vi "KioskDemo.vi"() -> ()   [LabVIEW 2023]
doc: "DESCRIPTION\nGeneral Application \n\nVERSION\nD1:00\nFirst Release To customer\nDD/MM/YYYY\n\nTemplate D2:01\nMade lighter and simpler\n14-04-2020"
uses:
  SubVIs/Controls/SetupModeState.ctl
  <vilib>/event_ctls.llb/eventsource.ctl
  <vilib>/Utility/miscctls.llb/LVBoundsTypeDef.ctl
  <vilib>/Utility/miscctls.llb/LVPositionTypeDef.ctl
  SubVIs/Controls/DisplayQCommand.ctl
  SubVIs/Controls/QueueCommand.ctl
  SubVIs/Controls/DisplayMessage.ctl
  SubVIs/Controls/Transition.ctl
  SubVIs/utilities/Error/ErrorCommand.ctl
  SubVIs/Controls/Tab.ctl
  SubVIs/Controls/StateMessage.ctl
  SubVIs/Error/ErrorMessage.ctl
  SubVIs/utilities/Config/System Config Data Manager Parameter.ctl
  SubVIs/utilities/Config/ConfigCommand.ctl
  SubVIs/Buttons/ButtonCommands.ctl
  SubVIs/Buttons/MenuType.ctl
panel:
  in  "ButtonsMenu":enum32{"Page 1"}(tab)
  out "SubmenuVisible":bool
  in  "Position":T1
  in  "Container Bounds":T2
  out "State":T3=enum."Initialising"
  out "UI Output":string
  out "Menu Output":string
  in  "exit":bool
  in  "Stop":bool
  in  "Source":T4 items=["LabVIEW UI"=0, "ActiveX"=1, "User Event"=25]
  out "Version":string
  out "Time":string
  in  "Main Screen Tabs":enum32{"Main Screen"}(tab)
  out "Tab Control":T5(tab)
  in  "Error Loop":enum16{"Event Loop", "UI Q Loop", "State Loop"}(ring)
  in  "Generate Error":bool
  out "EngMode?":bool
  in  "Enter Password":string
  out "ConfigdB path":path
  in  "Home Button":bool
  in  "ErrorLog":bool
  in  "Clear Alarm":bool
  in  "ErrorLog":i32(listbox)
  out "Error":string
  out "ErrorIndicator":bool
  in  "ViewError":bool
  out "Status":string
  in  "Start":bool
  out "ErrorHandlingLoop":i32
  out "StateMachineLoop":i32
  out "UILoop":i32
  out "EventLoop":i32
  # "GenAppMain"
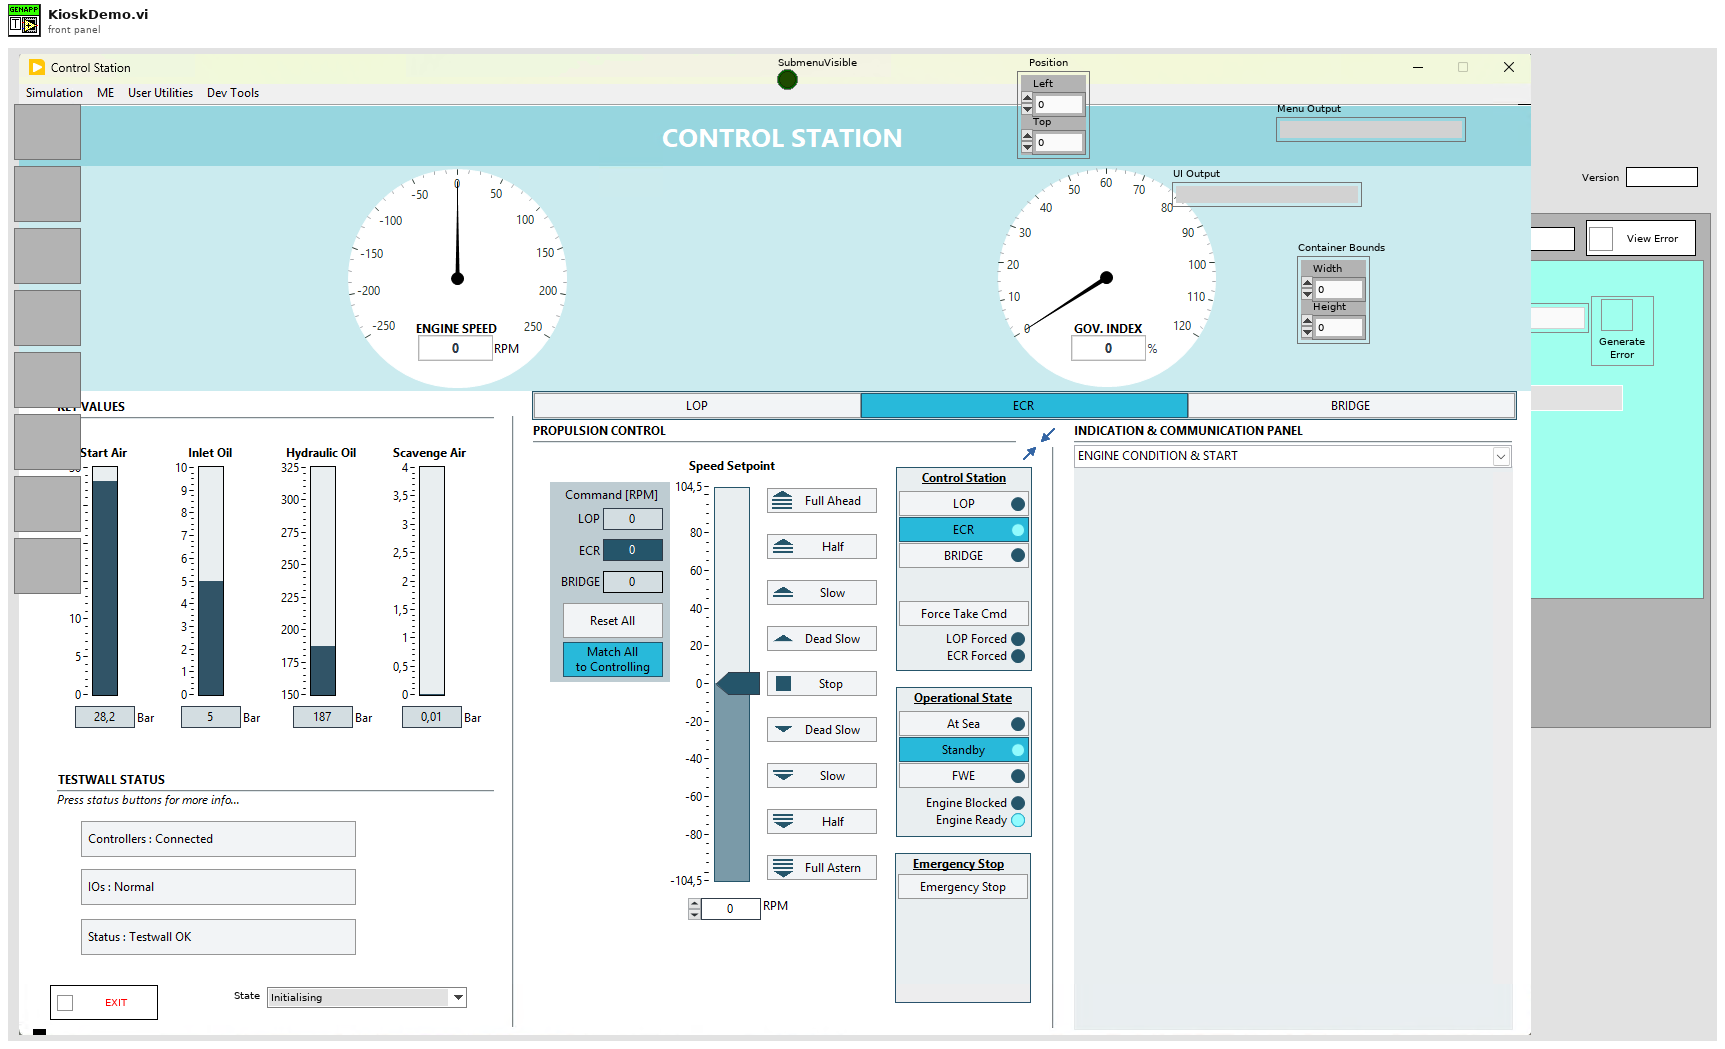
[diagram p1: front panel]
types:
  T1 = typedef "LVPositionTypeDef.ctl" = cluster{"Left":i32, "Top":i32}
  T2 = typedef "LVBoundsTypeDef.ctl" = cluster{"Width":u32, "Height":u32}
  T3 = typedef "SetupModeState.ctl" = enum16{"No State - Error", "Initialising", "Idling", "Running", "Sorting Menu", "Resetting Menu", "Loading UI", "Erroring", "Exiting"}
  T4 = typedef "eventsource.ctl" = u32
  T5 = enum32{"Welcome Screen", "Eng Set Up", "Oppo Run Screen", "Eng Run Screen", "Test Report Screen", "Error"}
  T6 = typedef "DisplayQCommand.ctl" = enum16{"No Command - Error", "Initialise", "Get Q Reference", "Add Item to Bottom", "Add Item to Top", "Flush Q", "Dequeue", "Peek Next Element", "Close"}
  T7 = typedef "QueueCommand.ctl" = enum16{"No Command - Error", "Initialise", "Add to Bottom", "Add To Top", "Get Ref", "Close"}
  T8 = typedef "ErrorCommand.ctl" = enum16{"No Command - Error", "Set to Dev Mode", "Set To Released Mode", "Set Error", "Log Error", "Throw Error", "Log & Throw Error", "Set Error Timed"}
  T9 = enum32{"invalid app kind", "Development System", "Run Time System", "Student Edition", "Embedded LabVIEW", "Evaluation", "Custom"}
  T10 = typedef "DisplayMessage.ctl" = enum16{"No Message - Ignore", "Display Message", "Set Tab", "Set Status", "Add Error Message", "Clear Error History", "Generate Error", "Set Idling Display", "Set Running Display", "Set Subpanel Output", "Stop"}
  T11 = typedef "ErrorMessage.ctl" = enum16{"No Message - Ignore", "Display Message", "Stop"}
  T12 = typedef "StateMessage.ctl" = cluster{"Transition":T13, "variant":variant}
  T13 = typedef "Transition.ctl" = enum16{"No Transition - Error", "Initialise", "Login", "Authenticate", "Log on Fail", "Login Success", "Logout", "Generate Error", "Start", "Stop", "Menu Button Pressed", "UI Button Pressed", "Exit"}
  T14 = typedef "ConfigCommand.ctl" = enum16{"No Command - Error", "Initialise Config SQLite", "Save Config", "Get Key", "Set Key", "Update Key", "Get Latest Config Data", "Get Config Data for Version", "Get Default Config Data"}
  T15 = typedef "System Config Data Manager Parameter.ctl" = enum16{"Eng Password", "DSN Connection", "User Password", "RunStatus", "InitialDataPath", "helpFilePath", "ErrorFilepath", "DatalogPath", "Hello"}
  T16 = typedef "Tab.ctl" = enum32{"Welcome Screen", "Eng Set Up", "Oppo Run Screen", "Eng Run Screen", "Test Report Screen", "Error"}
  T17 = typedef "lveventtype.ctl" = enum32{"Null", "Timeout", "Annotation Menu Selection", "Annotation Menu Selection?", "App Instance Close", "App Instance Close?", "Autoscale Range Change", "Bookmark Info Change", "Cell Edit", "Cell Edit?", "Cursor Grab", "Cursor Grab?", "Cursor Menu Selection", "Cursor Menu Selection?", "Cursor Move", "Cursor Release", "Data Change", "Direction Change", "Display State Change", "Drag Ended", "Drag Enter", "Drag Leave", "Drag Over", "Drag Source Update", "Drag Starting", "Drag Starting?", "Drop", "Exec State Change", "Key Down", "Key Down?", "Key Repeat", "Key Repeat?", "Key Up", "Listbox Double Click", "Menu Activation?", "Menu Selection (App)", "Menu Selection? (App)", "Menu Selection (User)", "Mouse Down", "Mouse Down?", "Mouse Enter", "Mouse Leave", "Mouse Move", "Mouse Up", "Mouse Wheel", "NI Security User Change (App)", "Pane Size", "Panel Close", "Panel Close?", "Panel Resize", "Plot Attribute Change", "Scale Range Change", "Shortcut Menu Activation?", "Shortcut Menu Selection (App)", "Shortcut Menu Selection? (App)", "Shortcut Menu Selection (User)", "Tree Double Click", "Tree Drag", "Tree Drag?", "Tree Drop", "Tree Drop?", "Tree Item Close", "Tree Item Close?", "Tree Item Open", "Tree Item Open?", "User Event", "Value Change"}
  T18 = typedef "MenuType.ctl" = enum16{"Main", "Simulation", "ME", "SF", "User Utilities", "Dev Tools"}
  T19 = typedef "ButtonCommands.ctl" = enum16{"No Command - Error", "Load Buttons", "Remove Buttons"}
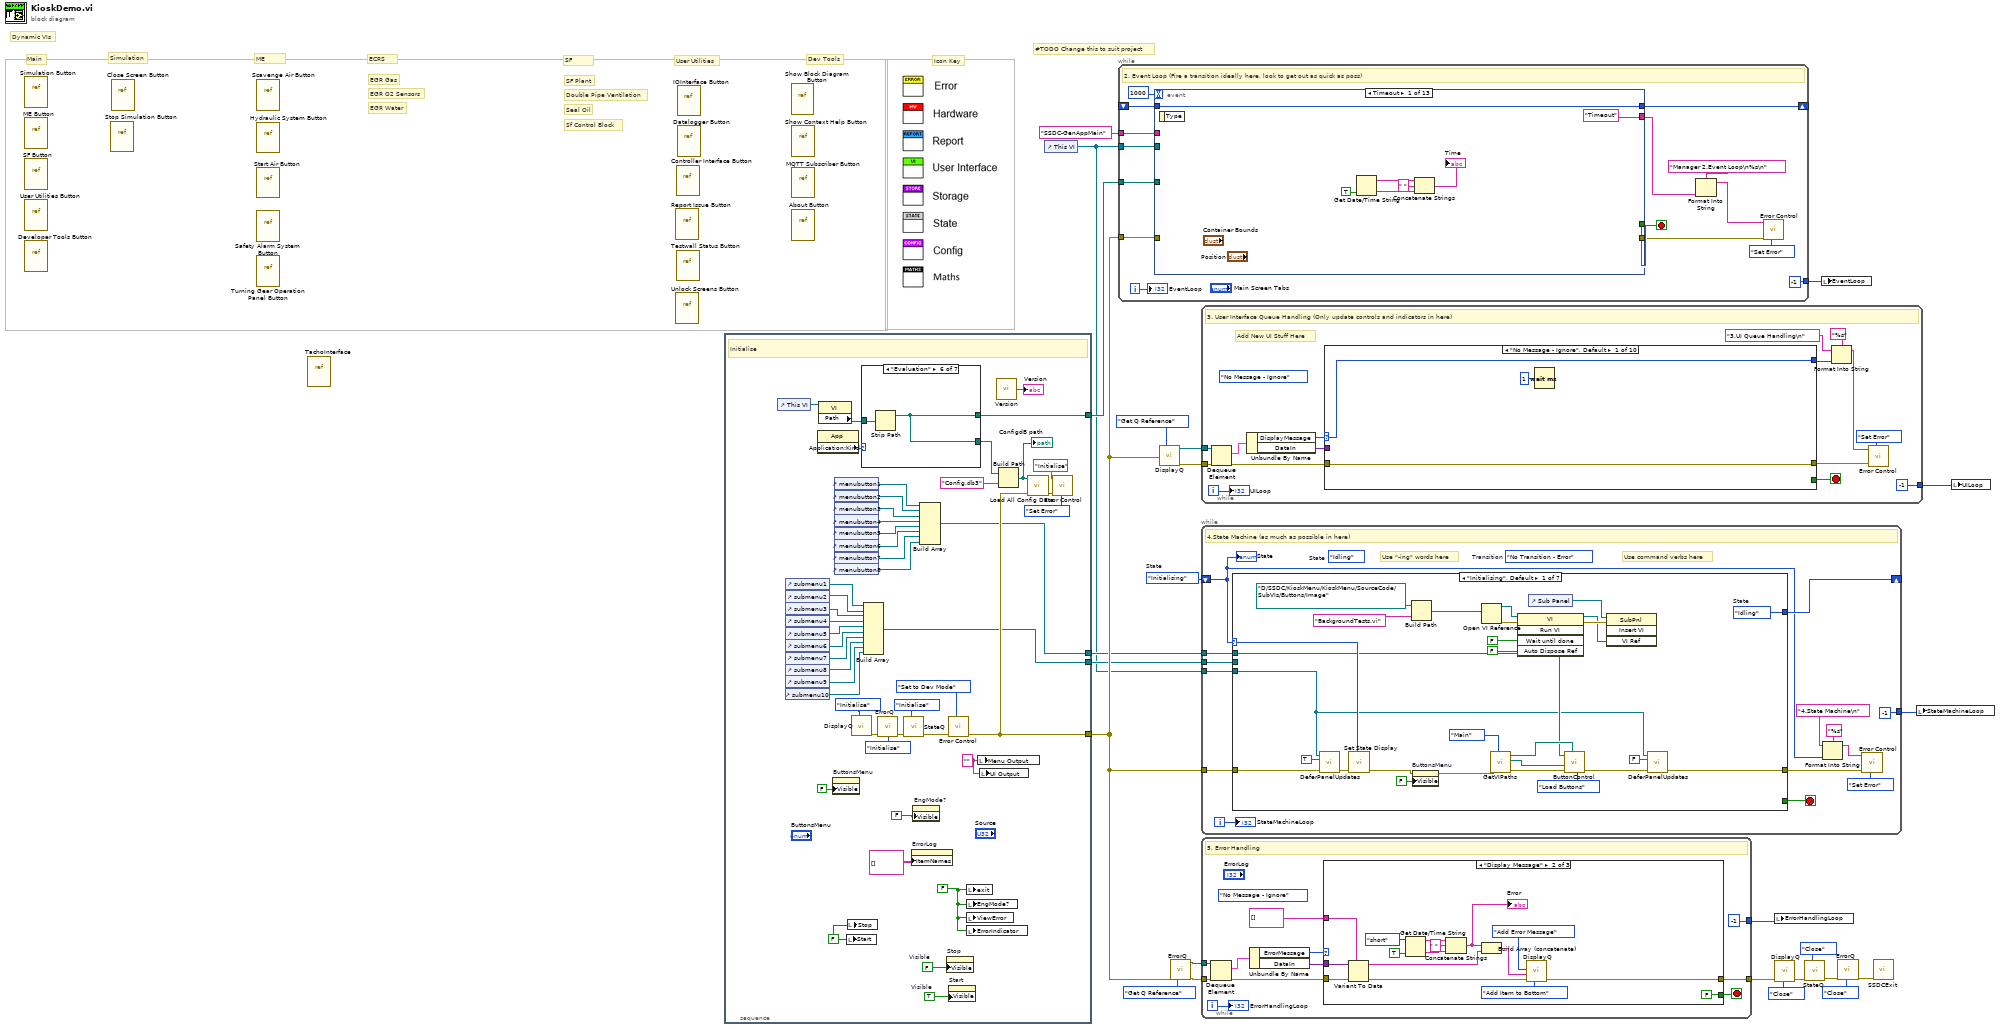
[diagram p0: block diagram]
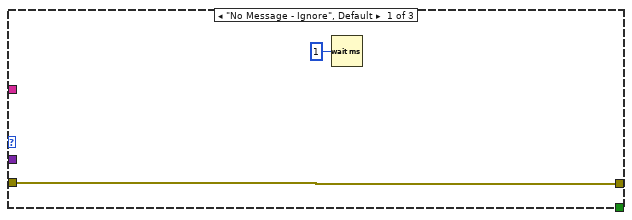
[diagram p2: hidden frame]
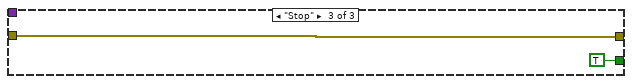
[diagram p3: hidden frame]
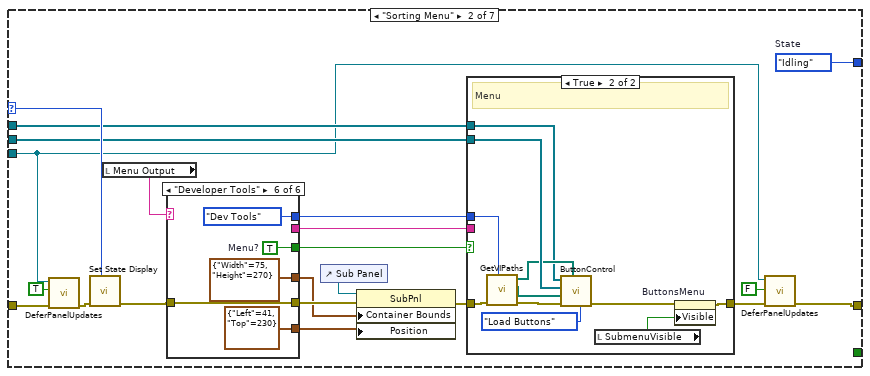
[diagram p4: hidden frame]
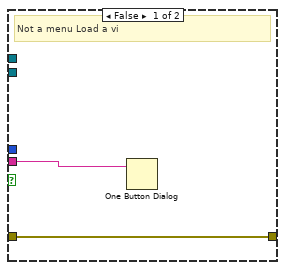
[diagram p5: hidden frame]
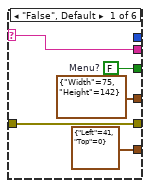
[diagram p6: hidden frame]
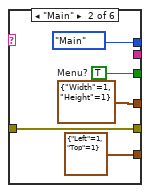
[diagram p7: hidden frame]
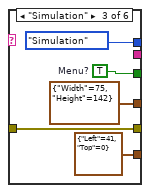
[diagram p8: hidden frame]
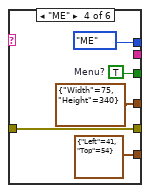
[diagram p9: hidden frame]
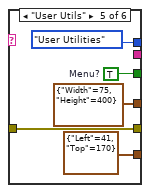
[diagram p10: hidden frame]
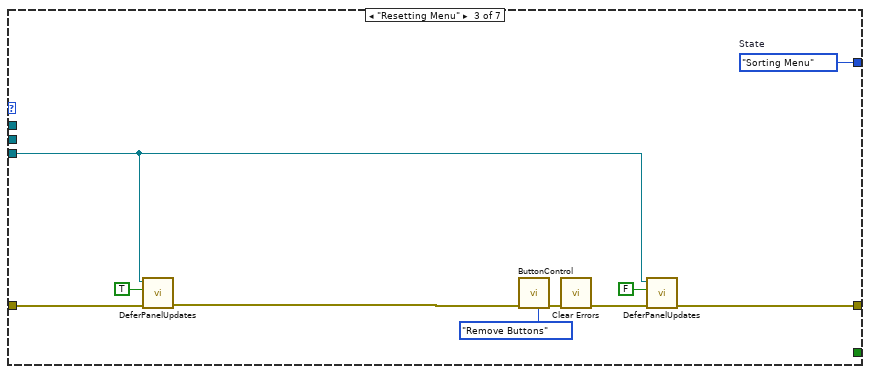
[diagram p11: hidden frame]
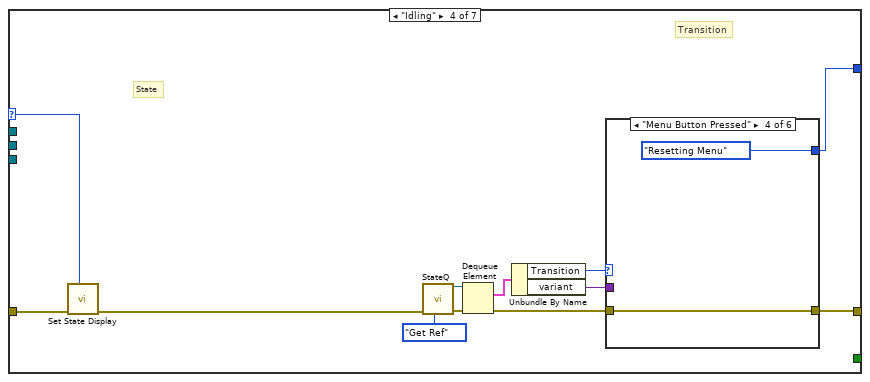
[diagram p12: hidden frame]
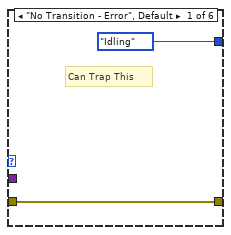
[diagram p13: hidden frame]
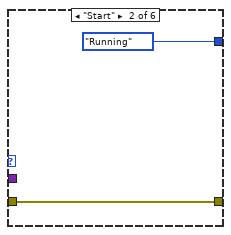
[diagram p14: hidden frame]
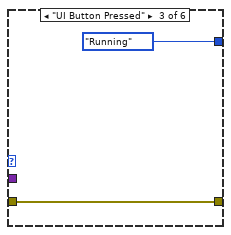
[diagram p15: hidden frame]
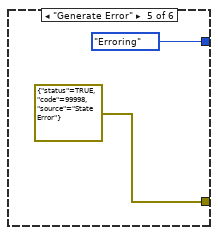
[diagram p16: hidden frame]
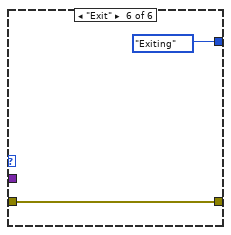
[diagram p17: hidden frame]
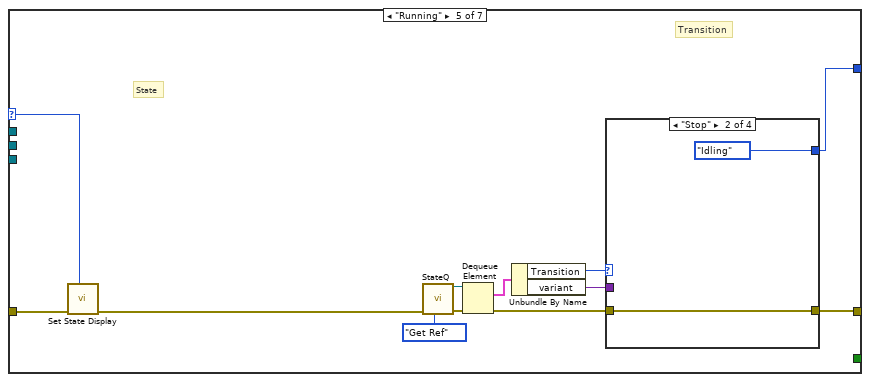
[diagram p18: hidden frame]
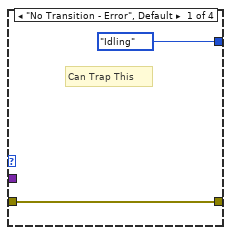
[diagram p19: hidden frame]
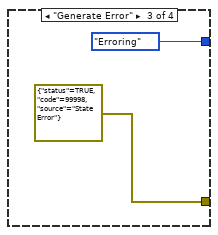
[diagram p20: hidden frame]
diagram:
  w24 = SetupModeState."Initialising"  # State
  # "Sf Control Block"
  # "Seal Oil"
  # "Double Pipe Ventilation"
  # "SF Plant"
  # "SF"
  # "EGR Water"
  # "EGR O2 Sensors"
  # "EGR Gas"
  # "ECRS"
  # "Dev Tools"
  # "User Utilities"
  # "Main"
  # "Simulation"
  # "ME"
  # "Dynamic VIs"
  # "#TODO Change this to suit project"
  # "Icon Key"
  n1 = vi-ref "Simulation Button.vi"() -> ()  [unwired: 1 out]
  n2 = vi-ref "ME Button.vi"() -> ()  [unwired: 1 out]
  n3 = vi-ref "SF Button.vi"() -> ()  [unwired: 1 out]
  n4 = vi-ref "User Utilities Button.vi"() -> ()  [unwired: 1 out]
  n5 = vi-ref "Developer Tools Button.vi"() -> ()  [unwired: 1 out]
  n6 = vi-ref "Stop Simulation Button.vi"() -> ()  [unwired: 1 out]
  n7 = vi-ref "Close Screen Button.vi"() -> ()  [unwired: 1 out]
  n8 = vi-ref "Scavenge Air Button.vi"() -> ()  [unwired: 1 out]
  n9 = vi-ref "Hydraulic System Button.vi"() -> ()  [unwired: 1 out]
  n10 = vi-ref "Start Air Button.vi"() -> ()  [unwired: 1 out]
  n11 = vi-ref "Safety Alarm System Button.vi"() -> ()  [unwired: 1 out]
  n12 = vi-ref "Turning Gear Operation Panel Button.vi"() -> ()  [unwired: 1 out]
  n13 = vi-ref "TachoInterface.vi"() -> ()  [unwired: 1 out]
  n14 = vi-ref "Report Issue Button.vi"() -> ()  [unwired: 1 out]
  n15 = vi-ref "Unlock Screens Button.vi"() -> ()  [unwired: 1 out]
  n16 = vi-ref "Controller Interface Button.vi"() -> ()  [unwired: 1 out]
  n17 = vi-ref "Testwall Status Button.vi"() -> ()  [unwired: 1 out]
  n18 = vi-ref "IOInterface Button.vi"() -> ()  [unwired: 1 out]
  n19 = vi-ref "Datalogger Button.vi"() -> ()  [unwired: 1 out]
  n20 = stacked-sequence "1. Initialisation" {
    tunnel: [w50] -> w11
    tunnel: [w55] -> w19
    tunnel: [w39] -> w3
    tunnel: [w31] -> w2
    frame #0 {
      w29 = "" ("Menu Output")
      w48 = FALSE  # Visible
      w47 = TRUE  # Visible
      w53 = FALSE ("Stopped")
      w49 = FALSE ("Start")
      # "Initialise"
      n21 = control-ref of="This VI"() -> (w66:refnum<vi>)
      n22 = control-ref of="submenu1"() -> (w38:refnum<vi>)
      n23 = control-ref of="submenu2"() -> (w37:refnum<vi>)
      n24 = control-ref of="submenu3"() -> (w36:refnum<vi>)
      n25 = control-ref of="submenu4"() -> (w35:refnum<vi>)
      n26 = control-ref of="submenu5"() -> (w34:refnum<vi>)
      n27 = control-ref of="submenu6"() -> (w33:refnum<vi>)
      n28 = control-ref of="submenu7"() -> (w32:refnum<vi>)
      n29 = control-ref of="submenu8"() -> (w28:refnum<vi>)
      n30 = control-ref of="submenu9"() -> (w27:refnum<vi>)
      n31 = control-ref of="submenu10"() -> (w26:refnum<vi>)
      n32 = property class="App"() -> ("Application:Kind"=w65:T9)  [unwired: 2 in, 2 out]
      n33 = property class="VI"(reference=w66) -> ("Path"=w67:path)  [unwired: 1 in, 2 out]
      n34 = property on="ButtonsMenu" class="TabCtl (strict)"("Visible"=FALSE) -> ()  [unwired: 2 in, 2 out]
      n35 = control-ref of="menubutton1"() -> (w41:refnum<vi>)
      n36 = control-ref of="menubutton2"() -> (w40:refnum<vi>)
      n37 = control-ref of="menubutton3"() -> (w46:refnum<vi>)
      n38 = control-ref of="menubutton4"() -> (w45:refnum<vi>)
      n39 = control-ref of="menubutton5"() -> (w44:refnum<vi>)
      n40 = control-ref of="menubutton6"() -> (w43:refnum<vi>)
      n41 = control-ref of="menubutton7"() -> (w42:refnum<vi>)
      n42 = control-ref of="menubutton8"() -> (w30:refnum<vi>)
      n43 = local write "Start"(w49) -> ()
      n44 = local write "Stop"(w49) -> ()
      n45 = call "DisplayQ.vi"("command"=DisplayQCommand."Initialise") -> ("error out"=w60:errorcluster)  [unwired: 4 in, 3 out]
      n46 = case shown="\"Evaluation\"" w65 {
        tunnel: w67 -> [w72 w74 w78 w81 w83 w85 w87]
        tunnel: [w72 w73 w77 w80 w82 w84 w86] -> w56
        tunnel: [w72 w73 w75 w80 w82 w84 w86] -> w55
        frame "invalid app kind", Default {
        }
        frame "Development System" {
          n47 = Strip Path(path=w74) -> (stripped path=w73:path)  [unwired: 1 out]
        }
        frame "Run Time System" {
          n48 = Strip Path(path=w78) -> (stripped path=w79:path)  [unwired: 1 out]
          n49 = Strip Path(path=w79) -> (stripped path=w75:path)  [unwired: 1 out]
          n50 = Build Path(base path=w75, name or relative path="data") -> (appended path=w77:path)
        }
        frame "Student Edition" {
          n51 = Strip Path(path=w81) -> (stripped path=w80:path)  [unwired: 1 out]
        }
        frame "Embedded LabVIEW" {
          n52 = Strip Path(path=w83) -> (stripped path=w82:path)  [unwired: 1 out]
        }
        frame "Evaluation" {
          n53 = Strip Path(path=w85) -> (stripped path=w84:path)  [unwired: 1 out]
        }
        frame "Custom" {
          n54 = Strip Path(path=w87) -> (stripped path=w86:path)  [unwired: 1 out]
        }
      }
      n55 = Build Array(w38, w37, w36, w35, w34, w33, w32, w28, w27, w26) -> (w31:refnum<vi>[])
      n56 = call "ErrorQ.vi"("command"=DisplayQCommand."Initialise", "error in (no error)"=w60) -> ("error out"=w61:errorcluster)  [unwired: 3 in, 3 out]
      n57 = call "StateQ.vi"("QueueCommand"=QueueCommand."Initialise", "error in (no error)"=w61) -> ("error out"=w51:errorcluster)  [unwired: 5 in, 1 out]
      n58 = property on="ErrorLog" class="MCListbox (strict)"("ItemNames"=string[][] [] ("Item Names")) -> ()  [unwired: 2 in, 2 out]
      n59 = property on="EngMode?" class="Bool (strict)"("Visible"=FALSE) -> ()  [unwired: 2 in, 2 out]
      n60 = Build Array(w41, w40, w46, w45, w44, w43, w42, w30) -> (w39:refnum<vi>[])
      n61 = property on="Stop" class="Bool (strict)"("Visible"=w48) -> ()  [unwired: 2 in, 2 out]
      n62 = call "Error Control.vi"("Command"=ErrorCommand."Set to Dev Mode", "error in (no error)"=w51) -> ("error out"=w50:errorcluster)  [unwired: 6 in]
      n63 = property on="Start" class="Bool (strict)"("Visible"=w47) -> ()  [unwired: 2 in, 2 out]
      n64 = local write "exit"(w53) -> ()
      n65 = local write "ViewError"(w53) -> ()
      n66 = local write "ErrorIndicator"(w53) -> ()
      n67 = local write "EngMode?"(w53) -> ()
      n68 = local write "Menu Output"(w29) -> ()
      n69 = local write "UI Output"(w29) -> ()
      n70 = call "Version.vi"() -> ("Version"=→"Version":string)  [unwired: 5 in]
      n71 = Build Path(base path=w56, name or relative path="Config.db3") -> (appended path=w68:path)
      "ConfigdB path" <- w68
      n72 = call "Load All Config Data.vi"("error in (no error)"=w50, "path"=w68) -> ("error out"=w58:errorcluster)  [unwired: 5 in]
      n73 = call "Error Control.vi"("Command"=ErrorCommand."Set Error", "error in (no error)"=w58, "Source"="Initialise") -> ()  [unwired: 5 in, 1 out]
    }
  }
  n74 = vi-ref "Show Block Diagram Button.vi"() -> ()  [unwired: 1 out]
  n75 = vi-ref "Show Context Help Button.vi"() -> ()  [unwired: 1 out]
  n76 = vi-ref "MQTT Subscriber Button.vi"() -> ()  [unwired: 1 out]
  n77 = vi-ref "About Button.vi"() -> ()  [unwired: 1 out]
  n78 = control-ref of="This VI"() -> (w1:refnum<vi>)
  n79 = while "2. Event Loop" {
    tunnel: w11 -> [w99]
    shift-right: [w96] -> _
    shift-left: _ -> [w95]
    tunnel: w1 -> [w94]
    tunnel: [-1 ("ErrorHandlingLoop")] -> w20
    tunnel: w19 -> [w92]
    tunnel: "SSDC-GenAppMain" ("name or relative path") -> [w91]
    i -> [w102]
    stop <- w101 stop-if-true
    # "2. Event Loop (Fire a transition ideally here, look to get out as quick as poss)"
    n80 = event shown="[0] Timeout" {
      selector: _ -> [_ _ _ _ _ _ _ _ _ _ _ _ _]
      dyn-events: _ -> [_ _ _ _ _ _ _ _ _ _ _ _ _]
      timeout: 1000 -> [_ _ _ _ _ _ _ _ _ _ _ _ _]
      tunnel: [_ FALSE ("STOP?") _ TRUE ("STOP?") _ _ _ w186 _ _ _ _ _] -> w101
      tunnel: w99 -> [_ w112 _ _ w144 w159 _ w183 w203 w221 w234 w257 _]
      tunnel: [_ w112 _ _ w143 w158 _ w182 w202 w220 w233 w256 _] -> w97
      tunnel: ["Timeout" "Panel Close?" ("Event") w116 w123 w140 w154 w168 w177 w195 w214 w227 w250 w269] -> w88
      tunnel: [w104 w111 w121 w126 w147 w161 w171 w185 w198 w219 w230 w258 w273] -> w96
      tunnel: w95 -> [w104 w111 w121 w126 w147 w161 w171 w185 _ w219 w230 w258 w273]
      tunnel: w94 -> [_ _ _ _ _ _ _ w184 _ _ _ _ w272]
      tunnel: w92 -> [_ _ _ _ _ _ _ w181 _ _ _ _ _]
      tunnel: w91 -> [_ _ _ _ _ _ _ _ _ _ _ _ _]
      event Timeout {
        n81 = event-data() -> ()  [unwired: 1 in, 1 out]
        n82 = Get Date/Time String(want seconds? (F)=TRUE) -> (date string=w108:string, time string=w107:string)  [unwired: 2 in]
        n83 = Concatenate Strings(w108, " " ("string"), w107) -> (→"Time":string)
      }
      event Panel Close? {
        n84 = event-data() -> ()  [unwired: 1 in, 1 out]
        n85 = property on="exit" class="Bool (strict)"("Val(Sgnl)"=TRUE ("Value (Signaling)")) -> ()  [unwired: 2 in, 2 out]
        n86 = event-data("Discard?"=TRUE) -> ()  [unwired: 1 in, 1 out]
      }
      event "ErrorLog": Value Change {
        n87 = event-data() -> ("CtlRef"=w118:refnum<vi>, "Type"=w117:T17)  [unwired: 1 in]
        n88 = call "CreateEventString.vi"("Type in"=w117, "Ctl Refnum"=w118) -> ("Event"=w116:string)  [unwired: 9 in]
        n89 = case shown="True" "ErrorLog" {
          tunnel: [_ FALSE] -> w119
          frame False {
          }
          frame True {
            n90 = call "ErrorLogDialog.vi"() -> ()  [unwired: 11 in, 1 out]
          }
        }
        n91 = local write "ErrorLog"(w119) -> ()
      }
      event "exit": Value Change {
        n92 = event-data() -> ("CtlRef"=w125:refnum<vi>, "Type"=w124:T17)  [unwired: 1 in]
        n93 = local write "Start"(FALSE ("Start")) -> ()
        n94 = call "CreateEventString.vi"("Type in"=w124, "Ctl Refnum"=w125) -> ("Event"=w123:string)  [unwired: 9 in]
        n95 = stacked-sequence {
          tunnel: [_ FALSE] -> w127
          frame #0 {
            n96 = call "StateQ.vi"("QueueCommand"=QueueCommand."Add To Top", "output cluster"=T12 {"Transition"=enum."Exit", "variant"=variant}) -> ("error out"=w134:errorcluster)  [unwired: 5 in, 1 out]
            n97 = call "ErrorQ.vi"("command"=DisplayQCommand."Add Item to Top", "error in (no error)"=w134, "ErrorMessage"=ErrorMessage."Stop") -> ("error out"=w131:errorcluster)  [unwired: 2 in, 3 out]
            n98 = call "DisplayQ.vi"("command"=DisplayQCommand."Add Item to Top", "error in (no error)"=w131, "DisplayMessage"=DisplayMessage."Stop") -> ()  [unwired: 2 in, 4 out]
          }
          frame #1 {
            n99 = Wait (ms)(milliseconds to wait=u32 500) -> ()  [unwired: 1 out]
          }
        }
        n100 = local write "exit"(w127) -> ()
      }
      event "Start": Value Change {
        n101 = event-data() -> ("CtlRef"=w142:refnum<vi>, "Type"=w141:T17)  [unwired: 1 in]
        n102 = call "CreateEventString.vi"("Type in"=w141, "Ctl Refnum"=w142) -> ("Event"=w140:string)  [unwired: 9 in]
        n103 = case shown="True" "Start" {
          tunnel: [_ FALSE ("Start")] -> w145
          tunnel: w144 -> [w148 w150]
          tunnel: [w148 w149] -> w143
          frame False {
          }
          frame True {
            n104 = call "StateQ.vi"("QueueCommand"=QueueCommand."Add To Top", "error in (no error)"=w150, "output cluster"=T12 {"Transition"=enum."Start", "variant"=variant}) -> ("error out"=w149:errorcluster)  [unwired: 4 in, 1 out]
          }
        }
        n105 = local write "Start"(w145) -> ()
      }
      event "Stop": Value Change {
        n106 = event-data() -> ("CtlRef"=w156:refnum<vi>, "Type"=w155:T17)  [unwired: 1 in]
        n107 = call "CreateEventString.vi"("Type in"=w155, "Ctl Refnum"=w156) -> ("Event"=w154:string)  [unwired: 9 in]
        n108 = case shown="True" "Stop" {
          tunnel: [_ FALSE ("Start")] -> w160
          tunnel: w159 -> [w162 w164]
          tunnel: [w162 w163] -> w158
          frame False {
          }
          frame True {
            n109 = call "StateQ.vi"("QueueCommand"=QueueCommand."Add To Top", "error in (no error)"=w164, "output cluster"=T12 {"Transition"=enum."Stop", "variant"=variant}) -> ("error out"=w163:errorcluster)  [unwired: 4 in, 1 out]
          }
        }
        n110 = local write "Stop"(w160) -> ()
      }
      event "Enter Password": Value Change {
        n111 = event-data() -> ("CtlRef"=w170:refnum<vi>, "Type"=w169:T17)  [unwired: 1 in]
        n112 = call "CreateEventString.vi"("Type in"=w169, "Ctl Refnum"=w170) -> ("Event"=w168:string)  [unwired: 9 in]
        n113 = call "SQLiteConfig.vi"("ConfigCommand"=ConfigCommand."Get Key", "Parameter"=System_Config_Data_Manager_Parameter."Eng Password") -> ("KeyData"=w172:string)  [unwired: 3 in, 3 out]
        n114 = Equal?(x=w172, y="Enter Password") -> (x = y?=w176:bool)
        "EngMode?" <- w176
        n115 = property on="EngMode?" class="Bool (strict)"("Visible"=w176) -> ()  [unwired: 2 in, 2 out]
      }
      event Menu Selection (User) {
        n116 = event-data() -> ("Type"=w179:T17, "ItemTag"=w178:string)  [unwired: 1 in]
        n117 = Format Into String(format string="\"Menu\":%s:%s", w179, w178) -> (resulting string=w177:string)  [unwired: 2 in, 1 out]
        n118 = case shown="\"About\"" w178 {
          tunnel: [_ FALSE _ _] -> w186
          tunnel: w184 -> [_ _ _ w194]
          tunnel: w183 -> [w187 w188 w191 w192]
          tunnel: [w187 w188 w191 w192] -> w182
          tunnel: w181 -> [_ _ _ _]
          frame "False", Default {
          }
          frame "Exit" {
            n119 = property on="exit" class="Bool (strict)"("Val(Sgnl)"=TRUE ("Value (Signaling)")) -> ()  [unwired: 2 in, 2 out]
          }
          frame "Configuration" {
            n120 = call "ConfigSQLiteSettingDialog.vi"() -> ()  [unwired: 1 in]
          }
          frame "About" {
            n121 = property class="VI"(reference=w194) -> ("Description"=w193:string)  [unwired: 1 in, 2 out]
            n122 = call "AboutScreen.vi"("Version Info. In"=w193) -> ()  [unwired: 11 in]
          }
        }
      }
      event "ViewError": Value Change {
        n123 = event-data() -> ("CtlRef"=w196:refnum<vi>, "Type"=w197:T17)  [unwired: 1 in]
        n124 = local read "Tab Control"() -> (w199:T5)
        n125 = call "CreateEventString.vi"("Type in"=w197, "Ctl Refnum"=w196) -> ("Event"=w195:string)  [unwired: 9 in]
        n126 = case shown="True" "ViewError" {
          tunnel: w203 -> [w206 w210]
          tunnel: [w206 w209] -> w202
          tunnel: [FALSE FALSE] -> w200
          tunnel: w199 -> [w204 w207]
          tunnel: [w204 w207] -> w198
          frame False {
          }
          frame True {
            n127 = call "DisplayQ.vi"("command"=DisplayQCommand."Add Item to Bottom", "error in (no error)"=w210, "DataIn"=Tab."Error" ("Tab Control"), "DisplayMessage"=DisplayMessage."Set Tab") -> ("error out"=w209:errorcluster)  [unwired: 1 in, 3 out]
          }
        }
        n128 = local write "ViewError"(w200) -> ()
      }
      event "Clear Alarm": Value Change {
        n129 = event-data() -> ("CtlRef"=w215:refnum<vi>, "Type"=w216:T17)  [unwired: 1 in]
        n130 = call "CreateEventString.vi"("Type in"=w216, "Ctl Refnum"=w215) -> ("Event"=w214:string)  [unwired: 9 in]
        n131 = case shown="True" "Clear Alarm" {
          tunnel: w221 -> [w223 w225]
          tunnel: [w223 w225] -> w220
          tunnel: [FALSE FALSE] -> w217
          frame False {
          }
          frame True {
            n132 = local write "ErrorIndicator"(FALSE ("ErrorIndicator")) -> ()
          }
        }
        n133 = local write "Clear Alarm"(w217) -> ()
      }
      event "Home Button": Value Change {
        n134 = event-data() -> ("CtlRef"=w229:refnum<vi>, "Type"=w228:T17)  [unwired: 1 in]
        n135 = call "CreateEventString.vi"("Type in"=w228, "Ctl Refnum"=w229) -> ("Event"=w227:string)  [unwired: 9 in]
        n136 = case shown="True" "Home Button" {
          tunnel: w234 -> [w236 w241]
          tunnel: [w236 w240] -> w233
          tunnel: [FALSE FALSE] -> w232
          tunnel: w230 -> [_ w238]
          frame False {
          }
          frame True {
            n137 = case shown="\"Error\"" w238 {
              tunnel: [Tab."Welcome Screen" ("Tab Control") Tab."Oppo Run Screen" ("Tab Control") Tab."Eng Run Screen" ("Tab Control") Tab."Test Report Screen" ("Tab Control") Tab."Error" ("Tab Control") Tab."Eng Run Screen" ("Tab Control")] -> w237
              frame "Welcome Screen" {
              }
              frame "Oppo Run Screen" {
              }
              frame "Eng Run Screen" {
              }
              frame "Test Report Screen" {
              }
              frame "Error" {
              }
              frame "Eng Set Up" {
              }
            }
            n138 = call "DisplayQ.vi"("command"=DisplayQCommand."Add Item to Bottom", "error in (no error)"=w241, "DataIn"=w237, "DisplayMessage"=DisplayMessage."Set Tab") -> ("error out"=w240:errorcluster)  [unwired: 1 in, 3 out]
          }
        }
        n139 = local write "Home Button"(w232) -> ()
      }
      event "Generate Error": Value Change {
        n140 = event-data() -> ("CtlRef"=w252:refnum<vi>, "Type"=w251:T17)  [unwired: 1 in]
        n141 = call "CreateEventString.vi"("Type in"=w251, "Ctl Refnum"=w252) -> ("Event"=w250:string)  [unwired: 9 in]
        n142 = case shown="\"UI Q Loop\"" "Error Loop" {
          tunnel: w257 -> [_ w261 w266]
          tunnel: [errorcluster {"status"=TRUE, "code"=99999, "source"="Random Event Error"} ("error out") w260 w267] -> w256
          tunnel: "Generate Error" -> [_ _ _]
          tunnel: [_ _ FALSE] -> w253
          frame "Event Loop", Default {
          }
          frame "UI Q Loop" {
            n143 = call "DisplayQ.vi"("command"=DisplayQCommand."Add Item to Bottom", "error in (no error)"=w261, "DisplayMessage"=DisplayMessage."Generate Error") -> ("error out"=w260:errorcluster)  [unwired: 2 in, 3 out]
          }
          frame "State Loop" {
            n144 = call "StateQ.vi"("QueueCommand"=QueueCommand."Add to Bottom", "error in (no error)"=w266, "output cluster"=T12 {"Transition"=enum."Generate Error", "variant"=variant}) -> ("error out"=w267:errorcluster)  [unwired: 4 in, 1 out]
          }
        }
        n145 = local write "Generate Error"(w253) -> ()
      }
      event "Version": Mouse Down {
        n146 = event-data() -> ("CtlRef"=w271:refnum<vi>, "Type"=w270:T17)  [unwired: 1 in]
        n147 = call "CreateEventString.vi"("Type in"=w270, "Ctl Refnum"=w271) -> ("Event"=w269:string)  [unwired: 9 in]
        n148 = property class="VI"(reference=w272) -> ("Description"=w274:string)  [unwired: 1 in, 2 out]
        n149 = call "VIDescription.vi"("VersionData In"=w274) -> ()  [unwired: 10 in, 1 out]
      }
    }
    n150 = Format Into String(format string="Manager 2.Event Loop\n%s\n", w88) -> (resulting string=w89:string)  [unwired: 2 in, 1 out]
    n151 = call "Error Control.vi"("Command"=ErrorCommand."Set Error", "error in (no error)"=w97, "Source"=w89) -> ()  [unwired: 5 in, 1 out]
    "EventLoop" <- w102
  }
  n152 = call "DisplayQ.vi"("command"=DisplayQCommand."Get Q Reference", "error in (no error)"=w11) -> ("error out"=w13:errorcluster, "queue out"=w14:refnum<queue>)  [unwired: 3 in, 2 out]
  n153 = call "ErrorQ.vi"("command"=DisplayQCommand."Get Q Reference", "error in (no error)"=w11) -> ("error out"=w16:errorcluster, "queue out"=w17:refnum<queue>)  [unwired: 3 in, 2 out]
  n154 = while {
    shift-right: [w286] -> _
    shift-left: w24 -> [w282]
    tunnel: w11 -> [w287]
    tunnel: [-1 ("ErrorHandlingLoop")] -> w22
    tunnel: w3 -> [w277]
    tunnel: w2 -> [w276]
    tunnel: w1 -> [w275]
    i -> [w285]
    stop <- w288 stop-if-true
    (unwired) SetupModeState."Idling"  # State
    (unwired) Transition."No Transition - Error"  # Transition
    # "Use command verbs here"
    # "Use \"-ing\" words here"
    # "4.State Machine (as much as possible in here)"
    n155 = case shown="\"Initialising\", Default" w282 {
      selector: w282 -> [w307 w336 _ w401 w425 w435 w446]
      tunnel: [_ _ _ _ _ _ TRUE] -> w288
      tunnel: w287 -> [w306 w323 w385 w402 w426 w439 w444]
      tunnel: [w316 w337 w390 w392 w416 w438 SetupModeState."No State - Error" ("State 2")] -> w286
      tunnel: [w305 w318 w384 w393 w417 w437 w443] -> w283
      tunnel: w277 -> [w304 w331 _ _ _ _ _]
      tunnel: w276 -> [_ w330 _ _ _ _ _]
      tunnel: w275 -> [w303 w317 w383 _ _ _ w445]
      frame "Initialising", Default {
        w316 = SetupModeState."Idling"  # State
        n156 = call "DeferPanelUpdates.vi"("error in (no error)"=w306, "Defer Panel Updates"=TRUE, "VI in"=w303) -> ("error out"=w310:errorcluster)  [unwired: 8 in]
        n157 = call "Set State Display.vi"("State"=w307, "error in (no error)"=w310) -> ("error out"=w300:errorcluster)  [unwired: 6 in]
        n158 = Build Path(base path=path "D:/SSDC/KioskMenu/KioskMenu/SourceCode/SubVIs/Buttons/Image" ("vi path"), name or relative path="BackgroundTests.vi") -> (appended path=w289:path)
        n159 = property on="ButtonsMenu" class="TabCtl (strict)"(error in=w300, "Visible"=FALSE) -> (error out=w299:errorcluster)  [unwired: 1 in, 1 out]
        n160 = Open VI Reference(vi path=w289) -> (vi reference=w295:refnum<vi>, error out=w296:errorcluster)  [unwired: 5 in]
        n161 = call "GetVIPaths.vi"("MenuType"=MenuType."Main", "error in (no error)"=w299) -> ("error out"=w315:errorcluster, "SubMenu VIs"=w313:path[], "Menu VIs"=w312:path[])  [unwired: 4 in]
        n162 = invoke class="VI" method="Run VI"(reference=w295, error in=w296, "Wait until done"=FALSE ("Wait Until Done"), "Auto Dispose Ref"=FALSE ("Auto Dispose Reference")) -> (reference out=w293:refnum<vi>, error out=w294:errorcluster)  [unwired: 1 in, 3 out]
        n163 = control-ref of="Sub Panel"() -> (w292:refnum<vi>)
        n164 = call "ButtonControl.vi"("SubPanel Command"=ButtonCommands."Load Buttons", "MenuButtons"=w312, "error in (no error)"=w315, "SubMenuButtons"=w313, "MenuButtonPanels"=w304) -> ("error out"=w308:errorcluster)  [unwired: 5 in]
        n165 = invoke on="Invoke Node" class="SubPnl" method="Insert VI"(reference=w292, error in=w294, "VI Ref"=w293) -> ()  [unwired: 1 in, 4 out]
        n166 = call "DeferPanelUpdates.vi"("error in (no error)"=w308, "Defer Panel Updates"=FALSE, "VI in"=w303) -> ("error out"=w305:errorcluster)  [unwired: 8 in]
      }
      frame "Sorting Menu" {
        w337 = SetupModeState."Idling"  # State
        n167 = call "DeferPanelUpdates.vi"("error in (no error)"=w323, "Defer Panel Updates"=TRUE, "VI in"=w317) -> ("error out"=w322:errorcluster)  [unwired: 8 in]
        n168 = call "Set State Display.vi"("State"=w336, "error in (no error)"=w322) -> ("error out"=w321:errorcluster)  [unwired: 6 in]
        n169 = local read "Menu Output"() -> (w335:string)
        n170 = case shown="\"Developer Tools\"" w335 {
          selector: w335 -> [w353 _ _ _ _ _]
          tunnel: w321 -> [w355 w360 w365 w370 w375 w380]
          tunnel: [w355 w360 w365 w370 w375 w380] -> w327
          tunnel: [_ MenuType."Main" ("MenuType") MenuType."Simulation" ("MenuType") MenuType."ME" ("MenuType") MenuType."User Utilities" ("MenuType") MenuType."Dev Tools" ("MenuType")] -> w334
          tunnel: [w354 w359 w364 w369 w374 w379] -> w333
          tunnel: [w353 _ _ _ _ _] -> w332
          tunnel: [T2 {"Width"=75, "Height"=142} ("Container Bounds") T2 {"Width"=1, "Height"=1} ("Container Bounds") T2 {"Width"=75, "Height"=142} ("Container Bounds") T2 {"Width"=75, "Height"=340} ("Container Bounds") T2 {"Width"=75, "Height"=400} ("Container Bounds") T2 {"Width"=75, "Height"=270} ("Container Bounds")] -> w326
          tunnel: [T1 {"Left"=41, "Top"=0} ("Position") T1 {"Left"=1, "Top"=1} ("Position") T1 {"Left"=41, "Top"=0} ("Position") T1 {"Left"=41, "Top"=54} ("Position") T1 {"Left"=41, "Top"=170} ("Position") T1 {"Left"=41, "Top"=230} ("Position")] -> w325
          frame "False", Default {
            w354 = FALSE  # Menu?
          }
          frame "Main" {
            w359 = TRUE  # Menu?
          }
          frame "Simulation" {
            w364 = TRUE  # Menu?
          }
          frame "ME" {
            w369 = TRUE  # Menu?
          }
          frame "User Utils" {
            w374 = TRUE  # Menu?
          }
          frame "Developer Tools" {
            w379 = TRUE  # Menu?
          }
        }
        n171 = control-ref of="Sub Panel"() -> (w329:refnum<vi>)
        n172 = property class="SubPnl"(reference=w329, error in=w327, "Container Bounds"=w326, "Position"=w325) -> (error out=w328:errorcluster)  [unwired: 1 out]
        n173 = case shown="True" w333 {
          tunnel: w328 -> [w339 w343]
          tunnel: [w339 w341] -> w319
          tunnel: w331 -> [_ w344]
          tunnel: w330 -> [_ w348]
          tunnel: w334 -> [_ w345]
          tunnel: w332 -> [w338 _]
          frame False {
            # "Not a menu Load a vi"
            n174 = One Button Dialog(message=w338) -> ()  [unwired: 1 in, 1 out]
          }
          frame True {
            # "Menu"
            n175 = call "GetVIPaths.vi"("MenuType"=w345, "error in (no error)"=w343) -> ("error out"=w350:errorcluster, "SubMenu VIs"=w347:path[], "Menu VIs"=w346:path[])  [unwired: 4 in]
            n176 = call "ButtonControl.vi"("SubPanel Command"=ButtonCommands."Load Buttons", "MenuButtons"=w346, "error in (no error)"=w350, "SubMenuButtons"=w347, "SubMenuButtonPanels"=w348, "MenuButtonPanels"=w344) -> ("error out"=w342:errorcluster)  [unwired: 4 in]
            n177 = local read "SubmenuVisible"() -> (w340:bool)
            n178 = property on="ButtonsMenu" class="TabCtl (strict)"(error in=w342, "Visible"=w340) -> (error out=w341:errorcluster)  [unwired: 1 in, 1 out]
          }
        }
        n179 = call "DeferPanelUpdates.vi"("error in (no error)"=w319, "Defer Panel Updates"=FALSE, "VI in"=w317) -> ("error out"=w318:errorcluster)  [unwired: 8 in]
      }
      frame "Resetting Menu" {
        w390 = SetupModeState."Sorting Menu"  # State
        n180 = call "DeferPanelUpdates.vi"("error in (no error)"=w385, "Defer Panel Updates"=TRUE, "VI in"=w383) -> ("error out"=w381:errorcluster)  [unwired: 8 in]
        n181 = call "ButtonControl.vi"("SubPanel Command"=ButtonCommands."Remove Buttons", "error in (no error)"=w381) -> ("error out"=w386:errorcluster)  [unwired: 8 in]
        n182 = call <vilib>:"Clear Errors.vi"("error in (no error)"=w386) -> ("error out"=w382:errorcluster)  [unwired: 5 in, 1 out]
        n183 = call "DeferPanelUpdates.vi"("error in (no error)"=w382, "Defer Panel Updates"=FALSE, "VI in"=w383) -> ("error out"=w384:errorcluster)  [unwired: 8 in]
      }
      frame "Idling" {
        # "Transition"
        # "State"
        n184 = call "Set State Display.vi"("State"=w401, "error in (no error)"=w402) -> ("error out"=w396:errorcluster)  [unwired: 6 in]
        n185 = call "StateQ.vi"("QueueCommand"=QueueCommand."Get Ref", "error in (no error)"=w396) -> ("error out"=w398:errorcluster, "queue out"=w397:refnum<queue>)  [unwired: 5 in]
        n186 = Dequeue Element(queue=w397, error in (no error)=w398) -> (element=w400:T12, error out=w395:errorcluster)  [unwired: 1 in, 2 out]
        n187 = Unbundle By Name(w400) -> ("Transition"=w394:T13, "variant"=w391:variant)
        n188 = case shown="\"Menu Button Pressed\"" w394 {
          tunnel: [SetupModeState."Idling" ("State 2") SetupModeState."Running" ("State 2") SetupModeState."Running" ("State 2") SetupModeState."Resetting Menu" ("State 2") SetupModeState."Erroring" ("State 2") SetupModeState."Exiting" ("State 2")] -> w392
          tunnel: w395 -> [w403 w405 w407 w409 _ w413]
          tunnel: [w403 w405 w407 w409 errorcluster {"status"=TRUE, "code"=99998, "source"="State Error"} ("error out") w413] -> w393
          tunnel: w391 -> [_ _ _ _ _ _]
          frame "No Transition - Error", Default {
            # "Can Trap This"
          }
          frame "Start" {
          }
          frame "UI Button Pressed" {
          }
          frame "Menu Button Pressed" {
          }
          frame "Generate Error" {
          }
          frame "Exit" {
          }
        }
      }
      frame "Running" {
        # "Transition"
        # "State"
        n189 = call "Set State Display.vi"("State"=w425, "error in (no error)"=w426) -> ("error out"=w420:errorcluster)  [unwired: 6 in]
        n190 = call "StateQ.vi"("QueueCommand"=QueueCommand."Get Ref", "error in (no error)"=w420) -> ("error out"=w422:errorcluster, "queue out"=w421:refnum<queue>)  [unwired: 5 in]
        n191 = Dequeue Element(queue=w421, error in (no error)=w422) -> (element=w424:T12, error out=w419:errorcluster)  [unwired: 1 in, 2 out]
        n192 = Unbundle By Name(w424) -> ("Transition"=w418:T13, "variant"=w415:variant)
        n193 = case shown="\"Stop\"" w418 {
          tunnel: [SetupModeState."Idling" ("State 2") SetupModeState."Idling" ("State 2") SetupModeState."Erroring" ("State 2") SetupModeState."Exiting" ("State 2")] -> w416
          tunnel: w419 -> [w427 w429 _ w433]
          tunnel: [w427 w429 errorcluster {"status"=TRUE, "code"=99998, "source"="State Error"} ("error out") w433] -> w417
          tunnel: w415 -> [_ _ _ _]
          frame "No Transition - Error", Default {
            # "Can Trap This"
          }
          frame "Stop" {
          }
          frame "Generate Error" {
          }
          frame "Exit" {
          }
        }
      }
      frame "Erroring" {
        # "Transition"
        # "State"
        n194 = call "Set State Display.vi"("State"=w435, "error in (no error)"=w439) -> ("error out"=w436:errorcluster)  [unwired: 6 in]
        n195 = call "WaitForTransition.vi"("error in (no error)"=w436, "State"=w435) -> ("error out"=w437:errorcluster, "StateOut"=w438:T3)  [unwired: 4 in]
      }
      frame "Exiting" {
        n196 = call "DeferPanelUpdates.vi"("error in (no error)"=w444, "Defer Panel Updates"=TRUE, "VI in"=w445) -> ("error out"=w449:errorcluster)  [unwired: 8 in]
        n197 = call "Set State Display.vi"("State"=w446, "error in (no error)"=w449) -> ("error out"=w441:errorcluster)  [unwired: 6 in]
        n198 = property on="ButtonsMenu" class="TabCtl (strict)"(error in=w441, "Visible"=FALSE) -> (error out=w440:errorcluster)  [unwired: 1 in, 1 out]
        n199 = call "ButtonControl.vi"("SubPanel Command"=ButtonCommands."Remove Buttons", "error in (no error)"=w440) -> ("error out"=w447:errorcluster)  [unwired: 8 in]
        n200 = call "DeferPanelUpdates.vi"("error in (no error)"=w447, "Defer Panel Updates"=FALSE, "VI in"=w445) -> ("error out"=w443:errorcluster)  [unwired: 8 in]
      }
    }
    n201 = Format Into String(format string="%s", initial string="4.State Machine\n", w282) -> (resulting string=w281:string)  [unwired: 1 in, 1 out]
    n202 = call "Error Control.vi"("Command"=ErrorCommand."Set Error", "error in (no error)"=w283, "Source"=w281) -> ()  [unwired: 5 in, 1 out]
    "StateMachineLoop" <- w285
    "State" <- w282
  }
  n203 = while {
    tunnel: w16 -> [w464]
    tunnel: w17 -> [w463]
    tunnel: [w455] -> w4
    tunnel: [-1 ("ErrorHandlingLoop")] -> w23
    i -> [w457]
    stop <- w458 stop-if-true
    (unwired) DisplayMessage."No Message - Ignore" ("DisplayMessage")
    # "5. Error Handling"
    n204 = Dequeue Element(queue=w463, error in (no error)=w464) -> (element=w462:cluster{"ErrorMessage":T11, "DataIn":variant}, error out=w459:errorcluster)  [unwired: 1 in, 2 out]
    n205 = Unbundle By Name(w462) -> ("ErrorMessage"=w460:T11, "DataIn"=w461:variant)
    n206 = case shown="\"Display Message\"" w460 {
      tunnel: w461 -> [_ w481 _]
      tunnel: w459 -> [w465 w480 w484]
      tunnel: [w465 w471 w484] -> w455
      tunnel: [_ FALSE ("STOP?") TRUE ("STOP?")] -> w458
      tunnel: string[] [] -> [_ w479 _]
      frame "No Message - Ignore", Default {
        n207 = Wait (ms)(milliseconds to wait=u32 1) -> ()  [unwired: 1 out]
      }
      frame "Display Message" {
        n208 = Variant To Data(error in=w480, type=w479, Variant=w481) -> (data=w473:string[], error out=w472:errorcluster)
        n209 = Get Date/Time String(date format (0)=enum16{"short", "long", "abbreviated"}."short", want seconds? (F)=TRUE) -> (date string=w476:string, time string=w475:string)  [unwired: 1 in]
        n210 = Concatenate Strings(w476, " " ("string"), w475) -> (w467:string)
        "Error" <- w467
        n211 = Build Array (concatenate)(w467, w473) -> (w468:string[])
        n212 = call "DisplayQ.vi"("command"=DisplayQCommand."Add Item to Bottom", "error in (no error)"=w472, "DataIn"=w468, "DisplayMessage"=DisplayMessage."Add Error Message") -> ("error out"=w471:errorcluster)  [unwired: 1 in, 3 out]
      }
      frame "Stop" {
      }
    }
    "ErrorHandlingLoop" <- w457
  }
  n213 = while "3. User Interface Queue Handling" {
    tunnel: w13 -> [w499]
    tunnel: w14 -> [w498]
    tunnel: [-1 ("ErrorHandlingLoop")] -> w21
    i -> [w490]
    stop <- w491 stop-if-true
    (unwired) DisplayMessage."No Message - Ignore" ("DisplayMessage")
    # "Add New UI Stuff Here"
    # "3. User Interface Queue Handling (Only update controls and indicators in here)"
    n214 = Dequeue Element(queue=w498, error in (no error)=w499) -> (element=w497:cluster{"DisplayMessage":T10, "DataIn":variant}, error out=w494:errorcluster)  [unwired: 1 in, 2 out]
    n215 = Unbundle By Name(w497) -> ("DisplayMessage"=w495:T10, "DataIn"=w496:variant)
    n216 = case shown="\"No Message - Ignore\", Default" w495 {
      selector: w495 -> [w500 w503 w506 w521 w528 w532 w536 w538 w540 w560]
      tunnel: w496 -> [_ _ w515 w524 _ _ _ _ w544 w546]
      tunnel: w494 -> [w501 w505 w508 w523 w527 w531 w535 _ w542 w547]
      tunnel: [w501 w505 w507 w522 w527 w531 w535 errorcluster {"status"=TRUE, "code"=99997, "source"="UI Error"} ("error out") w541 w545] -> w493
      tunnel: [_ TRUE ("STOP?") _ _ _ _ _ _ _ _] -> w491
      tunnel: [w500 w503 w506 w521 w528 w532 w536 w538 w540 w560] -> w489
      frame "No Message - Ignore", Default {
        n217 = Wait (ms)(milliseconds to wait=u32 1) -> ()  [unwired: 1 out]
      }
      frame "Stop" {
      }
      frame "Display Message" {
        n218 = Variant To Data(error in=w508, type="" ("data"), Variant=w515) -> (data=w511:string, error out=w507:errorcluster)
        n219 = local read "State"() -> (w513:T3)
        n220 = Format Into String(w513) -> (resulting string=w512:string)  [unwired: 3 in, 1 out]
        n221 = Concatenate Strings(w512, " - " ("string"), w511) -> (→"Status":string)
      }
      frame "Add Error Message" {
        n222 = property on="ErrorLog" class="MCListbox (strict)"() -> ("ItemNames"=w519:string[][])  [unwired: 2 in, 2 out]
        n223 = Variant To Data(error in=w523, type=string[] [], Variant=w524) -> (data=w518:string[], error out=w522:errorcluster)
        n224 = Build Array (concatenate)(w519, w518) -> (w516:string[][])
        n225 = property on="ErrorLog" class="MCListbox (strict)"("ItemNames"=w516) -> ()  [unwired: 2 in, 2 out]
        "ErrorIndicator" <- TRUE ("ErrorIndicator")
      }
      frame "Set Idling Display" {
        w525 = FALSE  # Visible
        w526 = TRUE  # Visible
        n226 = property on="Stop" class="Bool (strict)"("Visible"=w525) -> ()  [unwired: 2 in, 2 out]
        n227 = property on="Start" class="Bool (strict)"("Visible"=w526) -> ()  [unwired: 2 in, 2 out]
      }
      frame "Set Running Display" {
        w529 = TRUE  # Visible
        w530 = FALSE  # Visible
        n228 = property on="Stop" class="Bool (strict)"("Visible"=w529) -> ()  [unwired: 2 in, 2 out]
        n229 = property on="Start" class="Bool (strict)"("Visible"=w530) -> ()  [unwired: 2 in, 2 out]
      }
      frame "Clear Error History" {
        n230 = property on="ErrorLog" class="MCListbox (strict)"("ItemNames"=string[][] []) -> ()  [unwired: 2 in, 2 out]
        n231 = local write "ErrorIndicator"(FALSE ("ErrorIndicator")) -> ()
      }
      frame "Generate Error" {
      }
      frame "Set Tab" {
        n232 = Variant To Data(error in=w542, type=Tab."Eng Run Screen" ("Tab Control"), Variant=w544) -> (data=→"Tab Control":T16, error out=w541:errorcluster)
      }
      frame "Set Subpanel Output" {
        n233 = Variant To Data(error in=w547, type="", Variant=w546) -> (data=w559:string, error out=w552:errorcluster)
        n234 = Match Pattern(string=w559, regular expression=":") -> (after substring=w558:string, offset past match=w554:i32)  [unwired: 1 in, 2 out]
        n235 = Less Than 0?(x=w554) -> (x < 0?=w555:bool)
        n236 = case shown="False" w555 {
          tunnel: w558 -> [w564 _]
          tunnel: [Transition."Menu Button Pressed" ("Transition") Transition."UI Button Pressed" ("Transition")] -> w556
          tunnel: [w563 w568] -> w557
          tunnel: w559 -> [_ w568]
          frame False {
            # "Menu"
            n237 = local read "Menu Output"() -> (w566:string)
            n238 = Equal?(x=w566, y=w564) -> (x = y?=w562:bool)
            n239 = Not(x=w562) -> (.not. x?=→"SubmenuVisible":bool)
            n240 = Select(t="Main", s=w562, f=w564) -> (s? t:f=w563:string)
            "Menu Output" <- w563
          }
          frame True {
            # "UI"
            "UI Output" <- w568
          }
        }
        n241 = Bundle By Name(cluster=T12 {"Transition"=enum."No Transition - Error", "variant"=variant} ("output cluster"), "Transition"=w556, "variant"=w557) -> (w553:T12)
        n242 = call "StateQ.vi"("QueueCommand"=QueueCommand."Add to Bottom", "error in (no error)"=w552, "output cluster"=w553) -> ("error out"=w545:errorcluster)  [unwired: 4 in, 1 out]
      }
    }
    n243 = Format Into String(format string="%s", initial string="3.UI Queue Handling\n", w489) -> (resulting string=w488:string)  [unwired: 1 in, 1 out]
    n244 = call "Error Control.vi"("Command"=ErrorCommand."Set Error", "error in (no error)"=w493, "Source"=w488) -> ()  [unwired: 5 in, 1 out]
    "UILoop" <- w490
  }
  n245 = local write "ErrorHandlingLoop"(w23) -> ()
  n246 = call "DisplayQ.vi"("command"=DisplayQCommand."Close", "error in (no error)"=w4) -> ("error out"=w6:errorcluster)  [unwired: 3 in, 3 out]
  n247 = call "StateQ.vi"("QueueCommand"=QueueCommand."Close", "error in (no error)"=w6) -> ("error out"=w8:errorcluster)  [unwired: 5 in, 1 out]
  n248 = local write "EventLoop"(w20) -> ()
  n249 = call "ErrorQ.vi"("command"=DisplayQCommand."Close", "error in (no error)"=w8) -> ("error out"=w9:errorcluster)  [unwired: 3 in, 3 out]
  n250 = call "SSDCExit.vi"("error in (no error)"=w9) -> ()  [unwired: 6 in, 1 out]
  n251 = local write "StateMachineLoop"(w22) -> ()
  n252 = local write "UILoop"(w21) -> ()
